vi "Tosca-Initialize.vi"(0 "Tosca":refnum<class "Parameters.lvclass">, 5 "State":T1, 7 "IPC":T3, 11 "error in (no error)":errorcluster) -> (4 "Tosca out":refnum<class "Parameters.lvclass">, 15 "error out":errorcluster)   [LabVIEW 2020]
uses:
  IPC VIs/Tosca-IPC.ctl
  Classes/Parameters/Parameters.lvclass
  Digital Input VIs/Tosca-DI Queue Data.ctl
  Digital Input VIs/Tosca-Input Event.ctl
  Digital Input VIs/Tosca-Input Criterion.ctl
  epl-vi-lib/Utility VIs/Type Defs/Logic State.ctl
  Typedefs/Tosca-Accumulator.ctl
  Typedefs/Tosca-State AODO.ctl
  Typedefs/Tosca-AO Runtime.ctl
  Typedefs/Tosca-DO Runtime.ctl
  epl-vi-lib/Signal Synthesis VIs/4th Generation/Classes/SignalManager/SignalManager.lvclass
  Typedefs/Tosca-Synapse Start Data.ctl
  IPC VIs/Tosca-Message.ctl
  IPC VIs/Tosca-Message Action.ctl
  Typedefs/Tosca-Thread Type.ctl
  Imaging VIs/Tosca-2P-Notifier Data.ctl
  Typedefs/Tosca-MATLAB Queue Data.ctl
  Visual Stim VIs/Tosca-Grating.ctl
  Visual Stim VIs/Tosca-Grating Type.ctl
  Typedefs/Tosca-File IO Notification.ctl
  Typedefs/Tosca-State.ctl
  Classes/Parameters/Parameters.lvclass/Parameters.ctl
  Classes/Parameters/Write ParamFile.vi
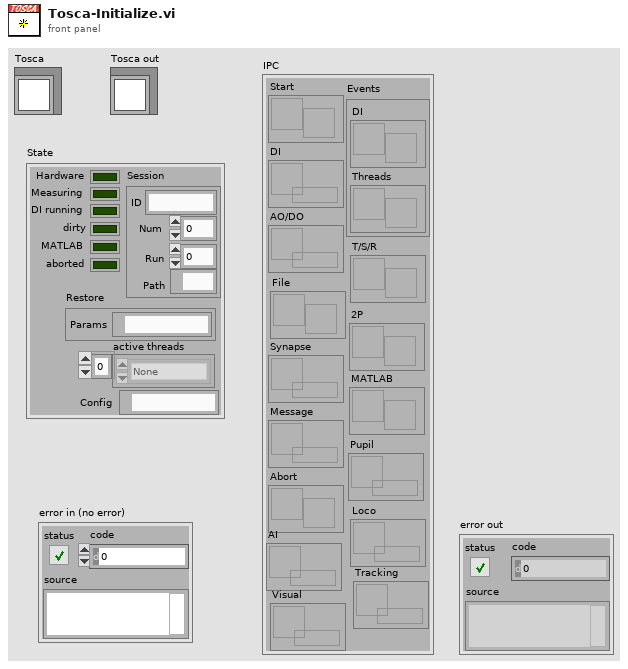
[diagram p1: front panel]
types:
  T1 = typedef "Tosca-State.ctl" = cluster{"Hardware":bool, "Measuring":bool, "DI running":bool, "dirty":bool, "Restore":cluster{"Params":path}, "Session":cluster{"ID":string, "Num":i32, "Path":path, "Run":i32}, "active threads":T2[], "MATLAB":bool, "Config":path, "aborted":bool}
  T2 = typedef "Tosca-Thread Type.ctl" = enum16{"None", "AODO", "Masker", "ET", "Imaging", "Pupil", "AI", "DI", "Camera", "TTL out", "Loco", "Visual"}
  T3 = typedef "Tosca-IPC.ctl" = cluster{"Start":refnum<notifier>, "DI":refnum<queue>, "AO/DO":refnum<queue>, "Synapse":refnum<queue>, "Message":refnum<queue>, "Abort":refnum<notifier>, "Events":cluster{"DI":refnum<user-event>, "Threads ":refnum<user-event>}, "T/S/R":refnum<notifier>, "2P":refnum<notifier>, "MATLAB":refnum<notifier>, "Pupil":refnum<queue>, "Loco":refnum<queue>, "AI":refnum<queue>, "Tracking":refnum<queue>, "Visual":refnum<queue>, "File":refnum<notifier>}
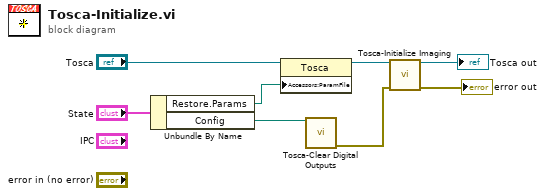
[diagram p0: block diagram]
diagram:
  n1 = Unbundle By Name("State") -> ("Restore.Params"=w5:path, "Config"=w6:path)
  n2 = property class="Tosca"(reference="Tosca", "Accessors:ParamFile"=w5) -> (reference out=w4:refnum<class "Parameters.lvclass">)  [unwired: 1 in, 1 out]
  n3 = call "Tosca-Clear Digital Outputs.vi"("Config path"=w6) -> ("error out"=w2:errorcluster)  [unwired: 14 in]
  n4 = call "Tosca-Initialize Imaging.vi"("Tosca"=w4, "error in (no error)"=w2) -> ("Tosca out"=→"Tosca out":refnum<class "Parameters.lvclass">, "error out"=→"error out":errorcluster)  [unwired: 12 in]
